vi "Creators Is Created Queue.vi"(10 "Created Queue Alias":string, 11 "Base Event in":refnum<class "Base Event.lvclass">) -> (2 "Is Created Queue?":bool, 3 "Base Event out":refnum<class "Base Event.lvclass">)   [LabVIEW 2021, in "jettl.lvlib" / "Base Event.lvlib" / "Base Event.lvclass"]
uses:
  Base Event.lvclass
  Queue Mailbox/Queue Mailbox.lvlib
  C:/git/jettl/jettl/jettl/jettl/jettl.lvclass
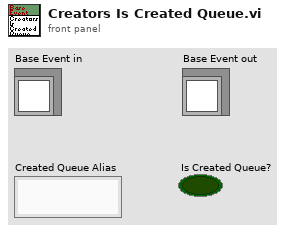
[diagram p1: front panel]
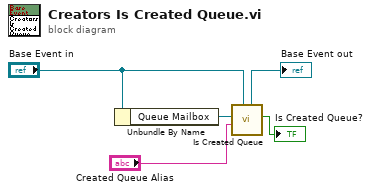
[diagram p0: block diagram]
diagram:
  n1 = Unbundle By Name("Base Event in") -> ("Queue Mailbox"=w5:refnum<data-value>)
  n2 = call "Is Created Queue.vi"("jettl in"="Base Event in", "Created Queue Alias"="Created Queue Alias", "Queue Mailbox"=w5) -> ("Is Created Queue?"=→"Is Created Queue?":bool, "jettl out"=→"Base Event out":refnum<class "Base Event.lvclass">)  [unwired: 7 in]
